vi "calculateTickPoints.vi"(8 "error in (no error)":errorcluster, 11 "PlayFile in":refnum<class "PlayFile.lvclass">) -> (0 "error out":errorcluster, 2 "TimeArray":dbl[](array[numeric]), 3 "PlayFile out":refnum<class "PlayFile.lvclass">)   [LabVIEW 2011, in "Tools.lvlib" / "Scripting.lvlib" / "PlayFile.lvclass"]
uses:
  PlayFile.lvclass
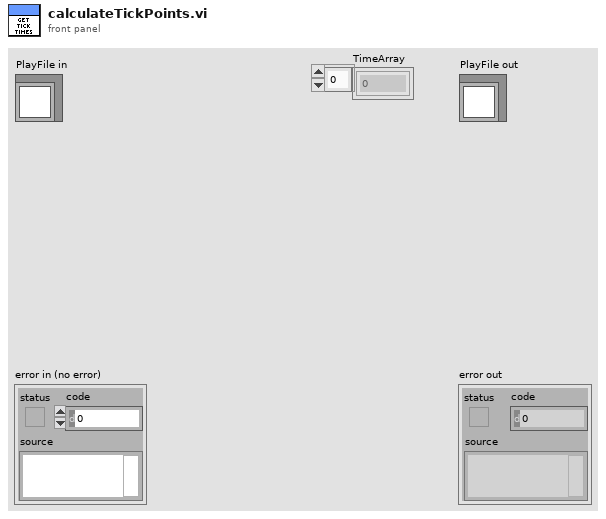
[diagram p1: front panel]
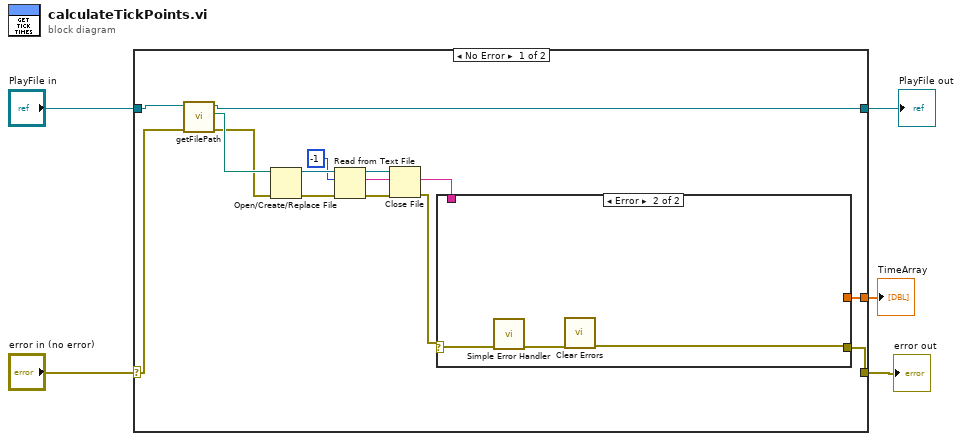
[diagram p0: block diagram]
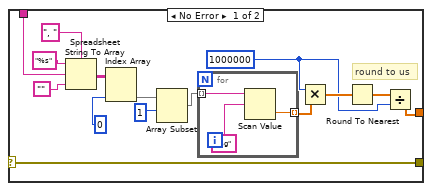
[diagram p2: hidden frame]
diagram:
  n1 = case shown="No Error" "error in (no error)" {
    selector: "error in (no error)" -> [w11 w42]
    tunnel: [w9 w42] -> w4
    tunnel: [w7 w41] -> w2
    tunnel: "PlayFile in" -> [w12 w41]
    tunnel: [w8 _] -> w1
    frame No Error {
      n2 = call "getFilePath.vi"("error in (no error)"=w11, "PlayFile in"=w12) -> ("error out"=w6:errorcluster, "filePath"=w10:path, "PlayFile out"=w7:refnum<class "PlayFile.lvclass">)  [unwired: 7 in]
      n3 = Open/Create/Replace File(file path (use dialog)=w10, error in=w6) -> (refnum out=w19:refnum<file>, error out=w18:errorcluster)  [unwired: 4 in, 1 out]
      n4 = Read from Text File(file (use dialog)=w19, count=-1, error in=w18) -> (refnum out=w16:refnum<file>, text=w14:string, error out=w17:errorcluster)  [unwired: 1 in, 1 out]
      n5 = Close File(refnum=w16, error in=w17) -> (error out=w13:errorcluster)  [unwired: 1 out]
      n6 = case shown="Error" w13 {
        selector: w13 -> [w29 w40]
        tunnel: w14 -> [w34 _]
        tunnel: [w29 w38] -> w9
        tunnel: [w23 _] -> w8
        frame No Error {
          w24 = 1000000
          # "round to us"
          n7 = Spreadsheet String To Array(delimiter (Tab)=", ", format string="%s", spreadsheet string=w34, array type (2D Dbl)="") -> (array=w28:string[][])
          n8 = Index Array(array=w28, index (col)=0 ("disabled index (col)")) -> (element=w20:string[])  [unwired: 1 in]
          n9 = Array Subset(array=w20, index=1) -> (w21:string[])  [unwired: 1 in]
          n10 = for {
            tunnel: w21 -> [w37] mode=indexing
            tunnel: [w35] -> w25 mode=indexing
            n11 = Scan Value(string=w37, format string="%g") -> (value=w35:dbl)  [unwired: 1 in, 1 out]
          }
          n12 = Multiply(x=w24, y=w25) -> (x*y=w27:dbl[])
          n13 = Round To Nearest(number=w27) -> (nearest integer value=w26:dbl[])
          n14 = Divide(x=w26, y=w24) -> (x/y=w23:dbl[])
        }
        frame Error {
          n15 = call <vilib>:"Simple Error Handler.vi"("error in (no error)"=w40) -> ("error out"=w39:errorcluster)  [unwired: 4 in, 4 out]
          n16 = call <vilib>:"Clear Errors.vi"("error in (no error)"=w39) -> ("error out"=w38:errorcluster)  [unwired: 6 in]
        }
      }
    }
    frame Error {
    }
  }
  "error out" <- w4
  "PlayFile out" <- w2
  "TimeArray" <- w1
